vi "Write Current Sense.vi"(8 "error in (no error)":errorcluster, 10 "Current Sense Engine Refs in":T1 {"RT IDs"."Slot #" max=15; "RT IDs"."Chip Address (A2 A1 A0)" max=7; "RT Block Data Refs"."Data Reference" format="%.0x"}, 11 "DMA FIFO Ref in":refnum<k20>) -> (0 "error out":errorcluster, 2 "Current Sense Engine Refs out":T1 {"RT IDs"."Slot #" max=15; "RT IDs"."Chip Address (A2 A1 A0)" max=7; "RT Block Data Refs"."Data Reference" format="%.0x"})   [LabVIEW 2014, in "SLSC configuration Engine.lvlib"]
uses:
  SLSC configuration Engine.lvlib
  Type Defs/RT Engine Refs.ctl
  Shared/Type Defs/RT IDs.ctl
  Shared/SPI Utility/Slot #.ctl
  Shared/MCP23S17/Chip Address.ctl
  <vilib>/NI Veristand/Custom Device API/Block Data Reference.ctl
  <vilib>/NI Veristand/Custom Device API/Data Reference.ctl
  <vilib>/NI Veristand/Custom Device API/Global Data Refs.vi
  <vilib>/NI Veristand/Custom Device API/Custom Device API.lvlib
  Shared/SLSC configuration Shared.lvlib
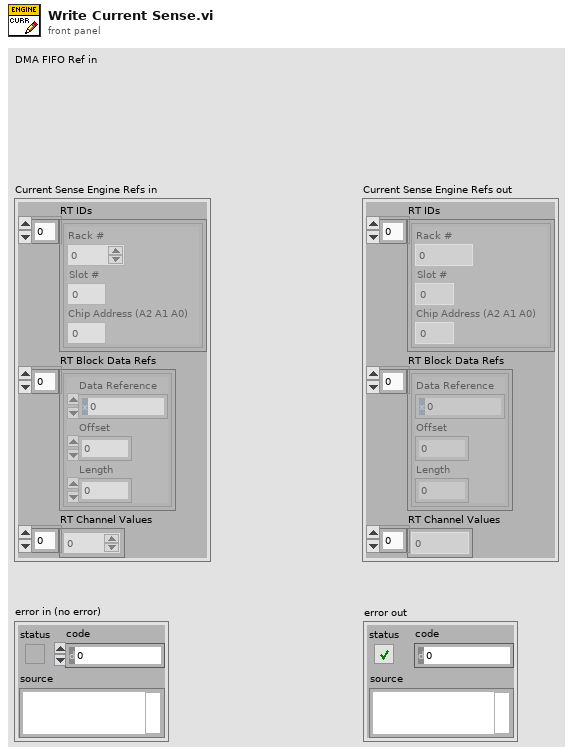
[diagram p1: front panel]
types:
  T1 = typedef "SLSC configuration Engine.lvlib/RT Engine Refs.ctl" = cluster{"RT IDs":T2[], "RT Block Data Refs":T5[], "RT Channel Values":dbl[]}
  T2 = typedef "SLSC configuration Shared.lvlib/RT IDs.ctl" = cluster{"Rack #":u8, "Slot #":T3, "Chip Address (A2 A1 A0)":T4}
  T3 = typedef "SLSC configuration Shared.lvlib/Slot #.ctl" = u8
  T4 = typedef "SLSC configuration Shared.lvlib/Chip Address.ctl" = u8
  T5 = typedef "Custom Device API.lvlib/Block Data Reference.ctl" = cluster{"Data Reference":T6, "Offset":i32, "Length":i32}
  T6 = typedef "Custom Device API.lvlib/Data Reference.ctl" = i32
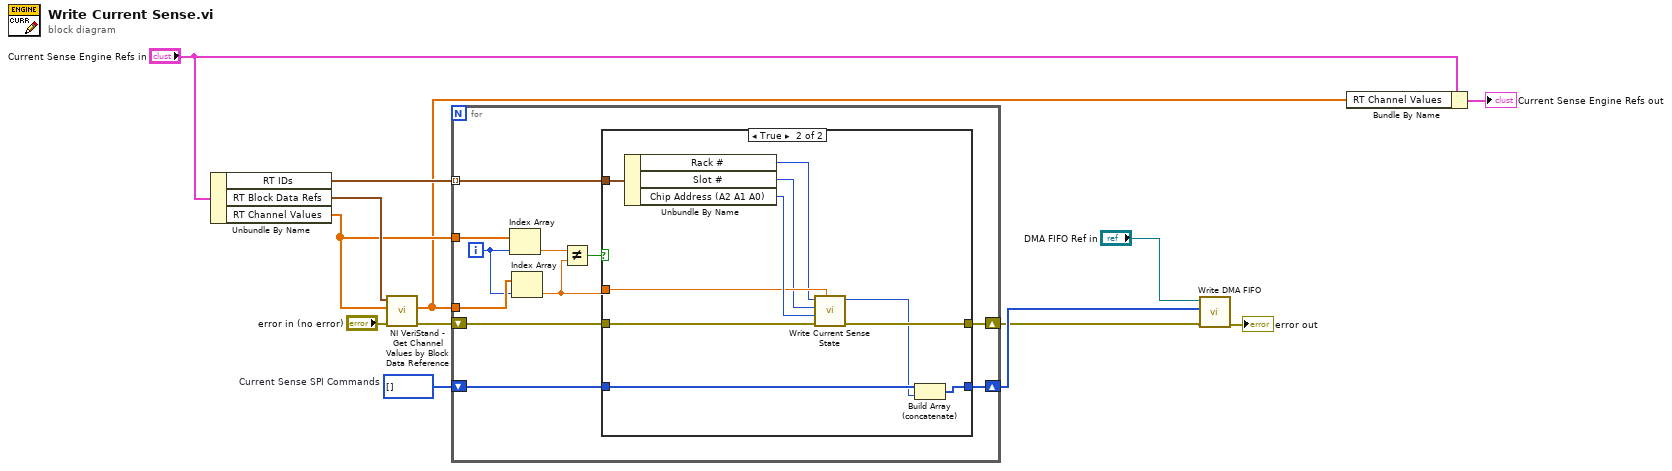
[diagram p0: block diagram]
diagram:
  w5 = u64[] []  # Current Sense SPI Commands
  n1 = Unbundle By Name("Current Sense Engine Refs in") -> ("RT IDs"=w10:T2[], "RT Block Data Refs"=w13:T5[], "RT Channel Values"=w8:dbl[])
  n2 = call <vilib>:"NI VeriStand - Get Channel Values by Block Data Reference.vi"("error in (no error)"="error in (no error)", "Values Array in"=w8, "Block Data Ref"=w13) -> ("error out"=w11:errorcluster, "Values Array out"=w7:dbl[])  [unwired: 6 in, 1 out]
  n3 = for {
    shift-right: [w18] -> w2
    shift-left: w11 -> [w20]
    tunnel: w10 -> [w21] mode=indexing
    tunnel: w7 -> [w23]
    tunnel: w8 -> [w24]
    shift-right: [w15] -> w3
    shift-left: w5 -> [w16]
    i -> [w14]
    n4 = Index Array(array=w24, index=w14) -> (element=w22:dbl)
    n5 = Index Array(array=w23, index=w14) -> (element=w19:dbl)
    n6 = Not Equal?(x=w22, y=w19) -> (x != y?=w17:bool)
    n7 = case shown="True" w17 {
      tunnel: w21 -> [_ w36]
      tunnel: w20 -> [w26 w35]
      tunnel: w19 -> [_ w29]
      tunnel: [w26 w33] -> w18
      tunnel: w16 -> [w25 w32]
      tunnel: [w25 w30] -> w15
      frame False {
      }
      frame True {
        n8 = Unbundle By Name(w36) -> ("Rack #"=w28:u8, "Slot #"=w27:T3, "Chip Address (A2 A1 A0)"=w34:T4)
        n9 = call "Write Current Sense State.vi"("Wheel Speed Sensor State"=w29, "error in (no error)"=w35, "Chip Address (A2 A1 A0)"=w34, "Slot #"=w27, "Rack #"=w28) -> ("error out"=w33:errorcluster, "FIFO SPI Message"=w31:u64)  [unwired: 4 in, 1 out]
        n10 = Build Array (concatenate)(w32, w31) -> (w30:u64[])
      }
    }
  }
  n11 = call "Write DMA FIFO.vi"("error in (no error)"=w2, "FIU SPI Commands"=w3, "DMA FIFO Ref in"="DMA FIFO Ref in") -> ("error out"=→"error out":errorcluster)  [unwired: 8 in]
  n12 = Bundle By Name(cluster="Current Sense Engine Refs in", "RT Channel Values"=w7) -> (→"Current Sense Engine Refs out":T1)
